vi "test_problems.vi"() -> ()   [LabVIEW 2018]
uses:
  <instrlib>/niDCPower/nidcpower.llb/niDCPower Source Mode.ctl
  <instrlib>/niDCPower/nidcpower.llb/niDCPower Output Function.ctl
panel:
  out "I2":dbl=-9.248393411097648e-06
  out "V2":dbl=0.000658308973496781
  out "I0":dbl=7.222553046148299e-05
  out "V0":dbl=-0.00030876303385435203
  out "Power off":bool=TRUE
  in  "POWER":bool
  in  "voltlim_I_LED, V":dbl=10.0 caption="current limit" min=0.01 format="%_6p"
  in  "I_LED, A":dbl=0.005 caption="voltage level" format="%_6p"
  in  "V_MB, V":dbl=5.0 caption="voltage level" format="%_6p"
  in  "curlim_V_MB, A":dbl=0.3 caption="current limit" format="%_6p"
  in  "curlim_V_RES, A":dbl=0.01 caption="current limit" min=0.01 format="%_6p"
  in  "V_RES, V":dbl=-1.0 caption="voltage level" format="%_6p"
  in  "current level range 1":dbl=0.001 caption="current level range" format="%#.6p"
  out "V1":dbl=0.0006698466238850311
  out "I1":dbl=-4.228096887639514e-06
  in  "Стоп":bool
  in  "Resource Name":refnum<k15>="PXI1Slot3" caption="Источник питания"
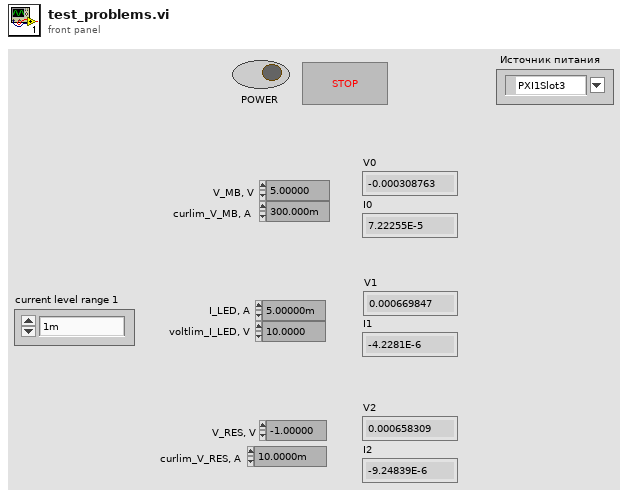
[diagram p1: front panel]
types:
  T1 = typedef "niDCPower Output Function.ctl" = i32
  T2 = typedef "niDCPower Source Mode.ctl" = i32
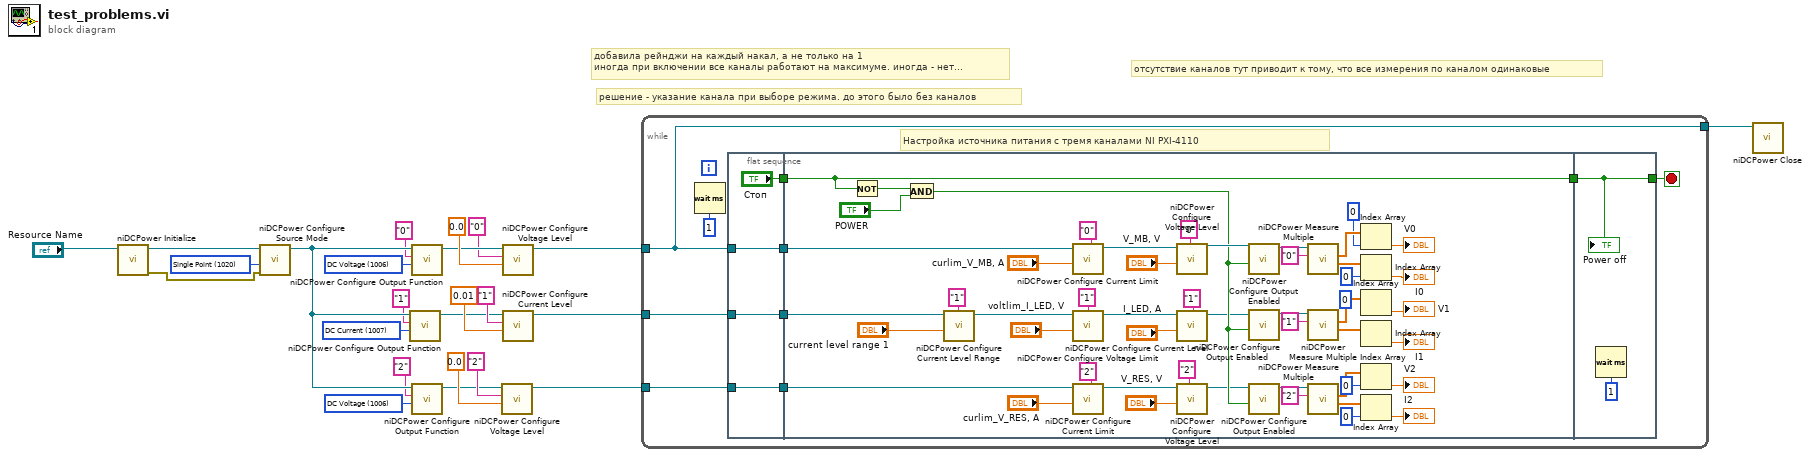
[diagram p0: block diagram]
diagram:
  w8 = T1 1006 items=["DC Voltage"=1006, "DC Current"=1007, "Pulse Voltage"=1049, "Pulse Current"=1050] ("output function")
  w15 = T1 1007 items=["DC Voltage"=1006, "DC Current"=1007, "Pulse Voltage"=1049, "Pulse Current"=1050] ("output function")
  w16 = T1 1006 items=["DC Voltage"=1006, "DC Current"=1007, "Pulse Voltage"=1049, "Pulse Current"=1050] ("output function")
  w19 = T2 1020 items=["Single Point"=1020, "Sequence"=1021] ("source mode")
  # "отсутствие каналов тут приводит к тому, что все измерения по каналом одинаковые"
  # "решение - указание канала при выборе режима. до этого было без каналов"
  # "добавила рейнджи на каждый накал, а не только на 1\nиногда при включении все каналы работают на максимуме. иногда - нет..."
  n1 = call <instrlib>:"niDCPower Initialize.vi"("resource name"="Resource Name") -> ("error out"=w5:errorcluster, "instrument handle out"=w20:refnum<k15>)  [unwired: 3 in, 6 out]
  n2 = call <instrlib>:"niDCPower Configure Source Mode.vi"("error in (no error)"=w5, "source mode"=w19, "instrument handle"=w20) -> ("instrument handle out"=w7:refnum<k15>)  [unwired: 8 out]
  n3 = call <instrlib>:"niDCPower Configure Output Function.vi"("output function"=w15, "channel name"="1", "instrument handle"=w7) -> ("instrument handle out"=w17:refnum<k15>)  [unwired: 7 in, 1 out]
  n4 = call <instrlib>:"niDCPower Configure Output Function.vi"("output function"=w16, "channel name"="0", "instrument handle"=w7) -> ("instrument handle out"=w18:refnum<k15>)  [unwired: 7 in, 1 out]
  n5 = call <instrlib>:"niDCPower Configure Output Function.vi"("output function"=w8, "channel name"="2", "instrument handle"=w7) -> ("instrument handle out"=w9:refnum<k15>)  [unwired: 7 in, 1 out]
  n6 = call <instrlib>:"niDCPower Configure Voltage Level.vi"("voltage level"=0.0, "channel name"="2", "instrument handle"=w9) -> ("instrument handle out"=w6:refnum<k15>)  [unwired: 7 in, 1 out]
  n7 = call <instrlib>:"niDCPower Configure Voltage Level.vi"("voltage level"=0.0, "channel name"="0", "instrument handle"=w18) -> ("instrument handle out"=w12:refnum<k15>)  [unwired: 7 in, 1 out]
  n8 = call <instrlib>:"niDCPower Configure Current Level.vi"("current level"=0.01, "channel name"="1", "instrument handle"=w17) -> ("instrument handle out"=w13:refnum<k15>)  [unwired: 7 in, 1 out]
  n9 = while {
    tunnel: w12 -> [w31]
    tunnel: [w31] -> w14
    tunnel: w13 -> [w28]
    tunnel: w6 -> [w25]
    stop <- w27 stop-if-true
    # "Настройка источника питания с тремя каналами NI PXI-4110"
    n10 = Wait (ms)(milliseconds to wait=u32 1) -> ()  [unwired: 1 out]
    n11 = flat-sequence {
      tunnel: w31 -> [w38]
      tunnel: [w38] -> w33
      tunnel: ["Стоп"] -> w32
      tunnel: [w36] -> w29
      tunnel: w28 -> [w36]
      tunnel: [w35] -> w26
      tunnel: w25 -> [w35]
      tunnel: w33 -> [w40]
      tunnel: w32 -> [w89]
      tunnel: [w89] -> w30
      tunnel: w29 -> [w57]
      tunnel: w26 -> [w39]
      tunnel: [w91] -> w27
      tunnel: w30 -> [w91]
      frame #0 {
      }
      frame #1 {
        n12 = Not(x=w89) -> (.not. x?=w88:bool)
        n13 = And(x=w88, y="POWER") -> (x .and. y?=w85:bool)
        n14 = call <instrlib>:"niDCPower Configure Current Level Range.vi"("current level range"="current level range 1", "channel name"="1", "instrument handle"=w57) -> ("instrument handle out"=w56:refnum<k15>)  [unwired: 7 in, 1 out]
        n15 = call <instrlib>:"niDCPower Configure Current Limit.vi"("current limit"="curlim_V_MB, A", "channel name"="0", "instrument handle"=w40) -> ("instrument handle out"=w77:refnum<k15>)  [unwired: 7 in, 1 out]
        n16 = call <instrlib>:"niDCPower Configure Voltage Limit.vi"("voltage limit"="voltlim_I_LED, V", "channel name"="1", "instrument handle"=w56) -> ("instrument handle out"=w81:refnum<k15>)  [unwired: 7 in, 1 out]
        n17 = call <instrlib>:"niDCPower Configure Current Limit.vi"("current limit"="curlim_V_RES, A", "channel name"="2", "instrument handle"=w39) -> ("instrument handle out"=w72:refnum<k15>)  [unwired: 7 in, 1 out]
        n18 = call <instrlib>:"niDCPower Configure Voltage Level.vi"("voltage level"="V_MB, V", "channel name"="0", "instrument handle"=w77) -> ("instrument handle out"=w86:refnum<k15>)  [unwired: 7 in, 1 out]
        n19 = call <instrlib>:"niDCPower Configure Current Level.vi"("current level"="I_LED, A", "channel name"="1", "instrument handle"=w81) -> ("instrument handle out"=w82:refnum<k15>)  [unwired: 7 in, 1 out]
        n20 = call <instrlib>:"niDCPower Configure Voltage Level.vi"("voltage level"="V_RES, V", "channel name"="2", "instrument handle"=w72) -> ("instrument handle out"=w73:refnum<k15>)  [unwired: 7 in, 1 out]
        n21 = call <instrlib>:"niDCPower Configure Output Enabled.vi"("output enabled"=w85, "instrument handle"=w86) -> ("instrument handle out"=w67:refnum<k15>)  [unwired: 8 in, 1 out]
        n22 = call <instrlib>:"niDCPower Configure Output Enabled.vi"("output enabled"=w85, "instrument handle"=w82) -> ("instrument handle out"=w60:refnum<k15>)  [unwired: 8 in, 1 out]
        n23 = call <instrlib>:"niDCPower Configure Output Enabled.vi"("output enabled"=w85, "instrument handle"=w73) -> ("instrument handle out"=w59:refnum<k15>)  [unwired: 8 in, 1 out]
        n24 = call <instrlib>:"niDCPower Measure Multiple.vi"("channel name"="0", "instrument handle"=w67) -> ("current measurements"=w65:dbl[], "voltage measurements"=w66:dbl[])  [unwired: 6 in, 2 out]
        n25 = call <instrlib>:"niDCPower Measure Multiple.vi"("channel name"="1", "instrument handle"=w60) -> ("current measurements"=w63:dbl[], "voltage measurements"=w64:dbl[])  [unwired: 6 in, 2 out]
        n26 = call <instrlib>:"niDCPower Measure Multiple.vi"("channel name"="2", "instrument handle"=w59) -> ("current measurements"=w61:dbl[], "voltage measurements"=w62:dbl[])  [unwired: 6 in, 2 out]
        n27 = Index Array(array=w66, index=0) -> (element=→"V0":dbl)
        n28 = Index Array(array=w65, index=0) -> (element=→"I0":dbl)
        n29 = Index Array(array=w64, index=0) -> (element=→"V1":dbl)
        n30 = Index Array(array=w63) -> (element=→"I1":dbl)  [unwired: 1 in]
        n31 = Index Array(array=w62, index=0) -> (element=→"V2":dbl)
        n32 = Index Array(array=w61, index=0) -> (element=→"I2":dbl)
      }
      frame #2 {
        n33 = Wait (ms)(milliseconds to wait=u32 1) -> ()  [unwired: 1 out]
        "Power off" <- w91
      }
    }
  }
  n34 = call <instrlib>:"niDCPower Close.vi"("instrument handle"=w14) -> ()  [unwired: 10 in, 1 out]
